vi "LDO Pressure Sensor to Burner ON_OFF.vi"(8 "error in (no error)":errorcluster, 11 "Sensor Data - LDO":string[][](array[string])=[["Water Inlet - Temperature (°F) - PL0001", "0.000000"], ["Water Outlet - Temperature (°F) - PL0002", "0.000000"], ["Ambient Temperature (°F)- PL0003", "0.000000"], ["Flue Exhaust Collector Box Top(°F)- PL0004", "0.000000"], ["Cold Supply Temperature (°F)- PL0005", "0.000000"], ["Hot Supply Temperature (°F)- PL0006", "0.000000"], ["TC Down (°F)- PL0007", "0.000000"], ["Ambient Temperature Outside Chamber (°F)- PL0008", "0.000000"], ["Flue Exhaust Collector Elbow (°F)- PL0009", "0.000000"], ["LDO Room Ceiling (°F)- PL0010", "0.000000"], ["Flue Gas Temperature (°F) - PL0011", "0.000000"], ["TC Type J (°F) - PL0012", "0.000000"], ["TC Type J (°F) - PL0013", "0.000000"], ["TC Type J (°F) - PL0014", "0.000000"], ["TC Type K (°F) - PL0015", "0.000000"], ["TC Type K (°F) - PL0016", "0.000000"], ["TC Type K (°F)- PL0017", "0.000000"], ["TC Type K (°F)- PL0018", "0.000000"], ["Blower Pressure (in W.C.)", "-1.000000"], ["Room Differential Pressure (in Water)", "-0.125000"], ["Gas Manifold Pressure (in Water)", "0"], ["Water Pressure Sensor (PSI)", "0.000000"], ["Flow Rate (GPM)", "0.000000"], ["Totalized Flow (Gallons)", "0.000000"], ["Counter of oil injections 0.8 cc/min", "0.000000"], ["Counter of oil injections 1.1 cc/min", "0.000000"], ["Counter of oil injections 1.33 cc/min", "0.000000"], ["Total Cycle Counter", "65535.000000"]]) -> (0 "error out":errorcluster, 3 "Burner ON?":bool)   [LabVIEW 2023]
panel:
  out "Manifold Pressure Data (in W.C)":string[](array[string])
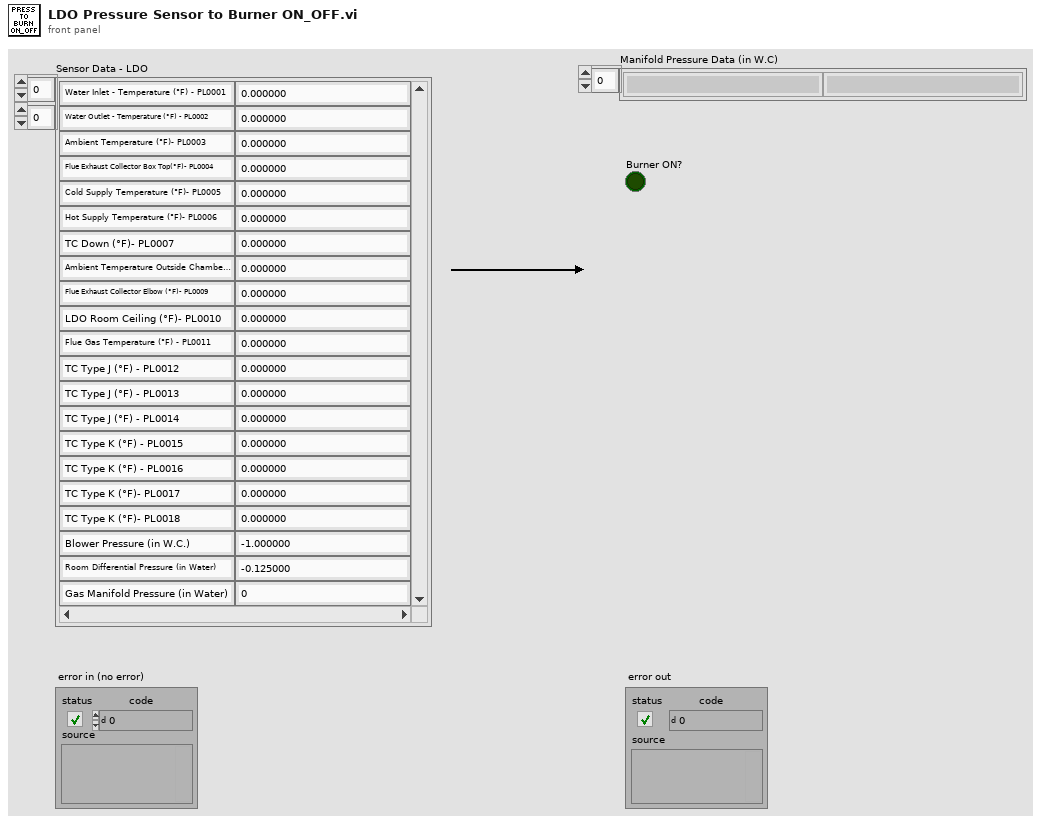
[diagram p1: front panel]
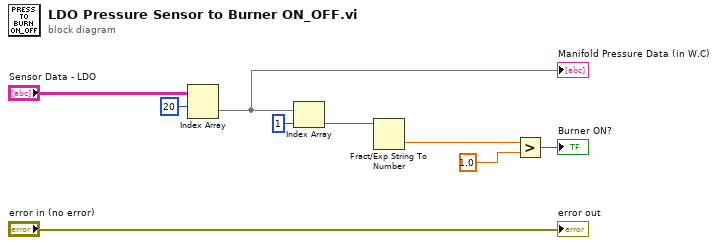
[diagram p0: block diagram]
diagram:
  n1 = Index Array(array="Sensor Data - LDO", index (row)=20) -> (element=w7:string[])  [unwired: 1 in]
  "Manifold Pressure Data (in W.C)" <- w7
  n2 = Index Array(array=w7, index=1) -> (element=w5:string)
  n3 = Fract/Exp String To Number(string=w5) -> (number=w4:dbl)  [unwired: 3 in, 1 out]
  n4 = Greater?(x=w4, y=1.0) -> (0:→"Burner ON?":bool)
  "error out" <- "error in (no error)"
